vi "stopShooting.vi"(8 "error in (no error)":errorcluster, 10 "stop":bool, 11 "ICCameraController in":refnum<class "ICCameraController.lvclass">) -> (0 "error out":errorcluster, 1 "Stopped":bool=TRUE, 2 "Array":path[](array[path]), 3 "ICCameraController out":refnum<class "ICCameraController.lvclass">)   [LabVIEW 2011, in "Hardware.lvlib" / "Channels.lvlib" / "ICCameraController.lvclass"]
uses:
  ICCameraController.lvclass
  ICCameraAcquisitor/ICCameraAcquisitor.lvclass
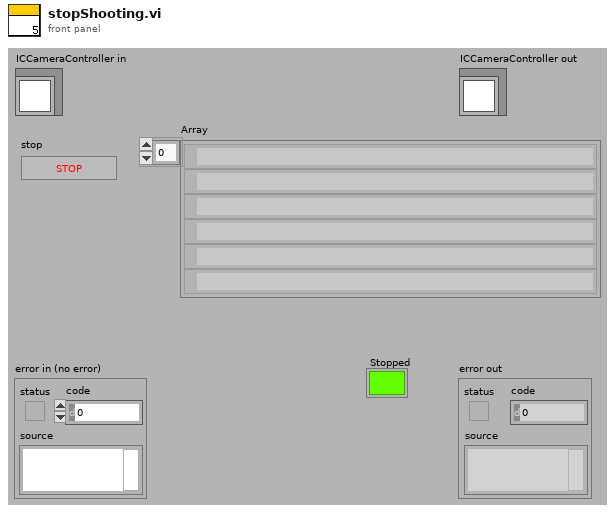
[diagram p1: front panel]
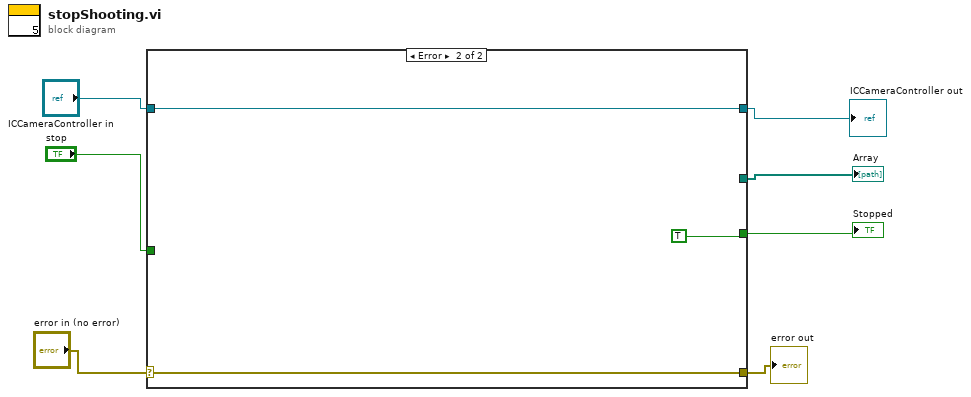
[diagram p0: block diagram]
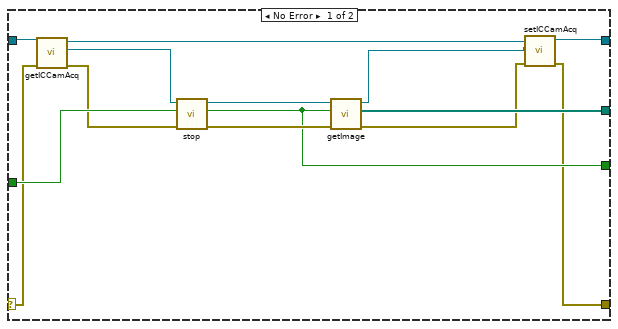
[diagram p2: hidden frame]
diagram:
  n1 = case shown="Error" "error in (no error)" {
    selector: "error in (no error)" -> [w14 w24]
    tunnel: [w8 w24] -> w4
    tunnel: [w11 w23] -> w1
    tunnel: "ICCameraController in" -> [w16 w23]
    tunnel: "stop" -> [w19 _]
    tunnel: [w17 TRUE] -> w3
    tunnel: [w18 _] -> w2
    frame No Error {
      n2 = call-dynamic "getICCamAcq.vi"("error in (no error)"=w14, "ICCameraController in"=w16) -> ("error out"=w13:errorcluster, "ICCameraAcquisitor"=w15:refnum<class "ICCameraAcquisitor.lvclass">, "ICCameraController out"=w12:refnum<class "ICCameraController.lvclass">)  [unwired: 7 in]
      n3 = call-dynamic "stop.vi"("error in (no error)"=w13, "Stop"=w19, "ICCameraAcquisitor in"=w15) -> ("error out"=w20:errorcluster, "Stopped"=w17:bool, "ICCameraAcquisitor out"=w21:refnum<class "ICCameraAcquisitor.lvclass">)  [unwired: 6 in]
      n4 = call-dynamic "getImage.vi"("error in (no error)"=w20, "stop"=w17, "ICCameraAcquisitor in"=w21) -> ("error out"=w9:errorcluster, "Array"=w18:path[], "ICCameraAcquisitor out"=w10:refnum<class "ICCameraAcquisitor.lvclass">)  [unwired: 6 in]
      n5 = call-dynamic "setICCamAcq.vi"("error in (no error)"=w9, "ICCameraAcquisitor"=w10, "ICCameraController in"=w12) -> ("error out"=w8:errorcluster, "ICCameraController out"=w11:refnum<class "ICCameraController.lvclass">)  [unwired: 7 in]
    }
    frame Error {
    }
  }
  "error out" <- w4
  "ICCameraController out" <- w1
  "Stopped" <- w3
  "Array" <- w2
